vi "Dashboard Code.vi"() -> ()   [LabVIEW 2015]
panel:
  out "New Image 4":T1(plugin-control)
  out "New Image 3":T1(plugin-control)
  out "New Image 2":T1(plugin-control)
  out "New Image":T1(plugin-control)
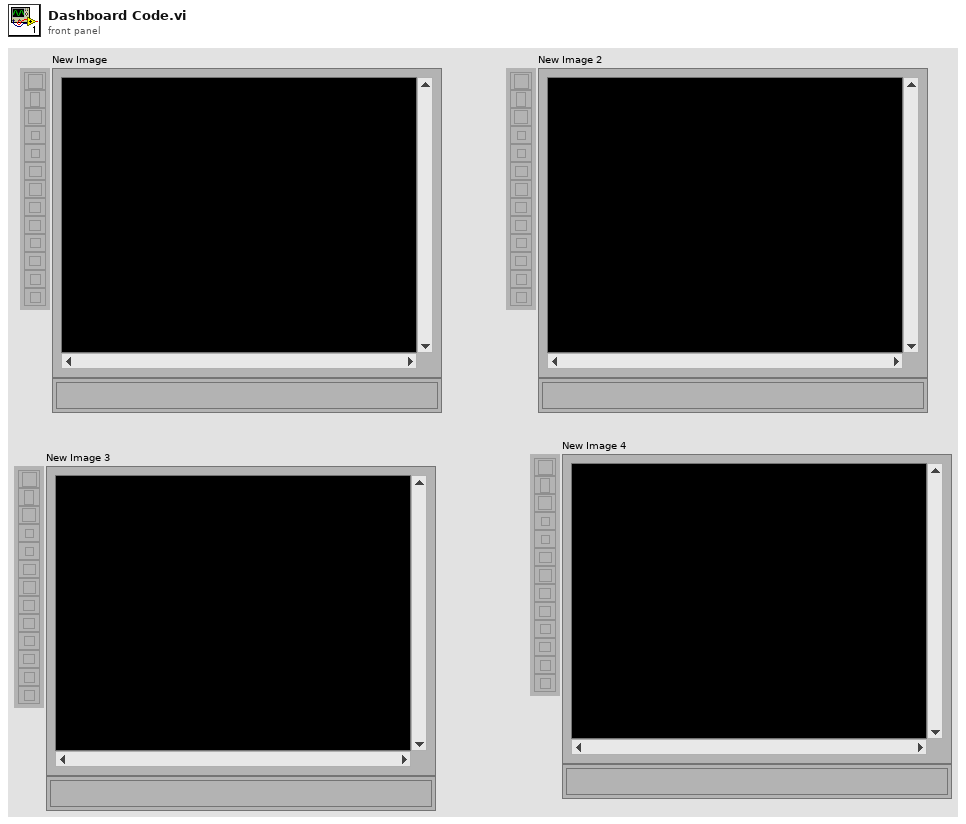
[diagram p1: front panel]
types:
  T1 = typedef "IMAQ Image.ctl" = refnum<image>
  T2 = cluster{"Camera Streams":i32, cluster{"occurrence":refnum<k4>, "New Image":T1}[]}
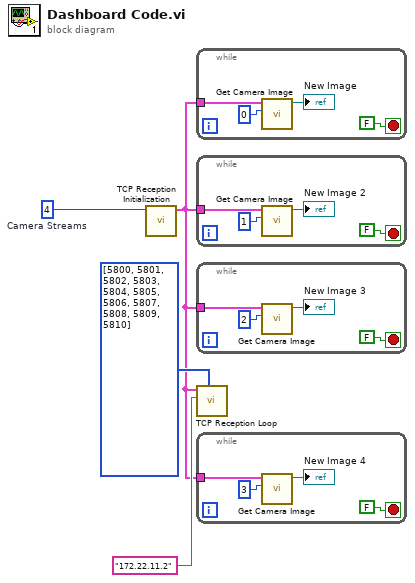
[diagram p0: block diagram]
diagram:
  w4 = 4  # Camera Streams
  n1 = call "TCP Reception Initialization.vi"("Camera Streams"=w4) -> ("Cluster"=w1:T2)  [unwired: 10 in]
  n2 = while {
    tunnel: w1 -> [w5]
    stop <- FALSE stop-if-true
    n3 = call "Get Camera Image.vi"("index"=0, "output cluster"=w5) -> ("Refnum out"=→"New Image":T1)  [unwired: 9 in]
  }
  n4 = while {
    tunnel: w1 -> [w9]
    stop <- FALSE stop-if-true
    n5 = call "Get Camera Image.vi"("index"=1, "output cluster"=w9) -> ("Refnum out"=→"New Image 2":T1)  [unwired: 9 in]
  }
  n6 = while {
    tunnel: w1 -> [w13]
    stop <- FALSE stop-if-true
    n7 = call "Get Camera Image.vi"("index"=2, "output cluster"=w13) -> ("Refnum out"=→"New Image 3":T1)  [unwired: 9 in]
  }
  n8 = call "TCP Reception Loop.vi"("Array 2"=u16[] [5800, 5801, 5802, 5803, 5804, 5805, 5806, 5807, 5808, 5809, 5810], "address"="172.22.11.2", "output cluster"=w1) -> ()  [unwired: 9 in]
  n9 = while {
    tunnel: w1 -> [w17]
    stop <- FALSE stop-if-true
    n10 = call "Get Camera Image.vi"("index"=3, "output cluster"=w17) -> ("Refnum out"=→"New Image 4":T1)  [unwired: 9 in]
  }
